vi "例程09-计算时间差.vi"() -> ()   [LabVIEW 2016]
panel:
  out "时间":dbl
  out "执行次数":i32
  out "随机产生的整数":u32
  in  "输入":u32
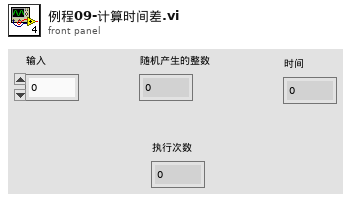
[diagram p1: front panel]
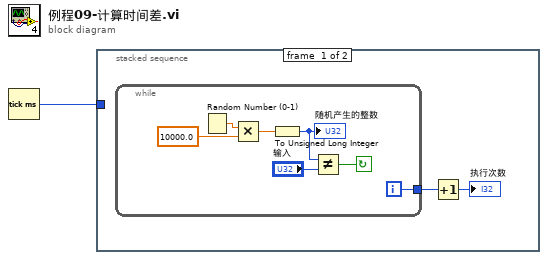
[diagram p0: block diagram]
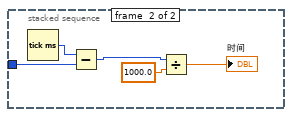
[diagram p2: hidden frame]
diagram:
  n1 = Tick Count (ms)() -> (millisecond timer value=w1:u32)
  n2 = stacked-sequence {
    tunnel: w1 -> [_ w12]
    frame #0 {
      n3 = while {
        tunnel: [w4] -> w3
        i -> [w4]
        stop <- w5 continue-if-true
        n4 = Random Number (0-1)() -> (number: 0 to 1=w10:dbl)
        n5 = Multiply(x=w10, y=10000.0) -> (x*y=w8:dbl)
        n6 = To Unsigned Long Integer(number=w8) -> (unsigned 32bit integer=w7:u32)
        "随机产生的整数" <- w7
        n7 = Not Equal?(x=w7, y="输入") -> (x != y?=w5:bool)
      }
      n8 = Increment(x=w3) -> (x+1=→"执行次数":i32)
    }
    frame #1 {
      n9 = Tick Count (ms)() -> (millisecond timer value=w11:u32)
      n10 = Subtract(x=w11, y=w12) -> (x-y=w15:u32)
      n11 = Divide(x=w15, y=1000.0) -> (x/y=→"时间":dbl)
    }
  }
